vi "Restore Panel by Section.vi"(8 "error in (no error)":errorcluster, 10 "VI reference":refnum<vi>, 11 "Path (dialog)":path=path "C:/ProgramData/EPL/CFTS Defaults.ini") -> (0 "Error Out":errorcluster)   [LabVIEW 2020]
doc: "Store the values in the controls of a front panel in a file.\n\nFreeware from Moore Good Ideas, www.mooregoodideas.com. Do not remove this line.\ndavid@mooregoodideas.com"
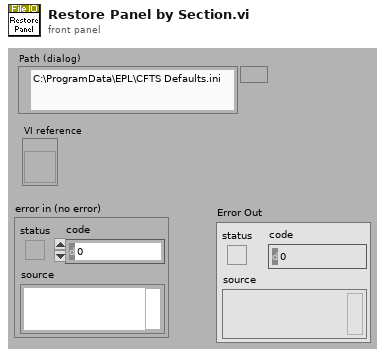
[diagram p1: front panel]
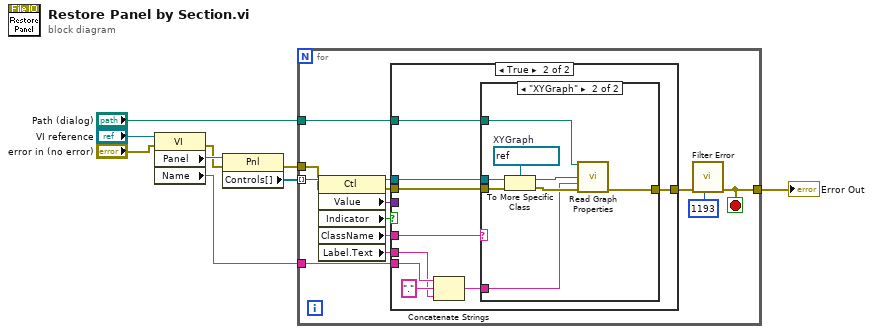
[diagram p0: block diagram]
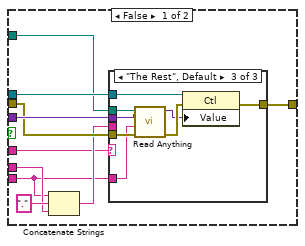
[diagram p2: hidden frame]
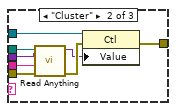
[diagram p4: hidden frame]
diagram:
  n1 = property class="VI"(reference="VI reference", error in="error in (no error)") -> (error out=w6:errorcluster, "Panel"=w7:refnum<vi>, "Name"=w1:string)  [unwired: 1 out]
  n2 = property class="Pnl"(reference=w7, error in=w6) -> (error out=w4:errorcluster, "Controls[]"=w5:refnum<vi>[])  [unwired: 1 out]
  n3 = for {
    tunnel: w5 -> [w22] mode=indexing
    tunnel: w4 -> [w21]
    tunnel: [w12] -> w3
    tunnel: "Path (dialog)" -> [w17]
    tunnel: w1 -> [w13]
    stop <- w12 stop-if-true
    n4 = property class="Ctl"(reference=w22, error in=w21) -> (reference out=w18:refnum<vi>, error out=w19:errorcluster, "Value"=w20:variant, "Indicator"=w16:bool, "ClassName"=w10:string, "Label.Text"=w14:string)
    n5 = case shown="True" w16 {
      tunnel: w20 -> [w32 _]
      tunnel: [w30 w50] -> w15
      tunnel: w19 -> [w28 w52]
      tunnel: w18 -> [w31 w53]
      tunnel: w17 -> [w29 w51]
      tunnel: w14 -> [w24 w56]
      tunnel: w13 -> [w23 w57]
      tunnel: w10 -> [w25 w55]
      frame False {
        n6 = Concatenate Strings(w23, "." ("string"), w24) -> (w26:string)
        n7 = case shown="\"The Rest\", Default" w25 {
          tunnel: w32 -> [_ w41 w49]
          tunnel: w31 -> [_ w40 w48]
          tunnel: [w33 w38 w46] -> w30
          tunnel: w29 -> [_ w36 w44]
          tunnel: w28 -> [w33 w35 w43]
          tunnel: w26 -> [_ w34 _]
          tunnel: w23 -> [_ _ w42]
          frame "" {
          }
          frame "Cluster" {
            n8 = call "Read Anything.vi"("Type of Anything"=w41, "Error In"=w35, "Section Name (Name of \"Type of Anything\")"=w34, "Path (dialog)"=w36) -> ("Error Out"=w39:errorcluster, "Anything"=w37:variant)  [unwired: 5 in, 1 out]
            n9 = property class="Ctl"(reference=w40, error in=w39, "Value"=w37) -> (error out=w38:errorcluster)  [unwired: 1 out]
          }
          frame "The Rest", Default {
            n10 = call "Read Anything.vi"("Type of Anything"=w49, "Error In"=w43, "Section Name (Name of \"Type of Anything\")"=w42, "Path (dialog)"=w44) -> ("Error Out"=w47:errorcluster, "Anything"=w45:variant)  [unwired: 5 in, 1 out]
            n11 = property class="Ctl"(reference=w48, error in=w47, "Value"=w45) -> (error out=w46:errorcluster)  [unwired: 1 out]
          }
        }
      }
      frame True {
        n12 = Concatenate Strings(w57, "." ("string"), w56) -> (w54:string)
        n13 = case shown="\"XYGraph\"" w55 {
          tunnel: w54 -> [_ w60]
          tunnel: w53 -> [_ w66]
          tunnel: w52 -> [w59 w65]
          tunnel: w51 -> [_ w64]
          tunnel: [w59 w61] -> w50
          frame "False", Default {
          }
          frame "XYGraph" {
            w67 = refnum<vi> refnum  # XYGraph
            n14 = To More Specific Class(target class=w67, reference=w66, error in=w65) -> (specific class reference=w63:refnum<vi>, error out=w62:errorcluster)
            n15 = call "Read Graph Properties.vi"("Config File"=w64, "WFGraph Refnum"=w63, "Section"=w60, "error in (no error)"=w62) -> ("error out"=w61:errorcluster)  [unwired: 10 in, 1 out]
          }
        }
      }
    }
    n16 = call "Filter Error.vi"("error in (no error)"=w15, "code to ignore"=1193) -> ("error out"=w12:errorcluster)  [unwired: 9 in]
  }
  "Error Out" <- w3
